vi "Tidy Project.vi"   [LabVIEW 2018]
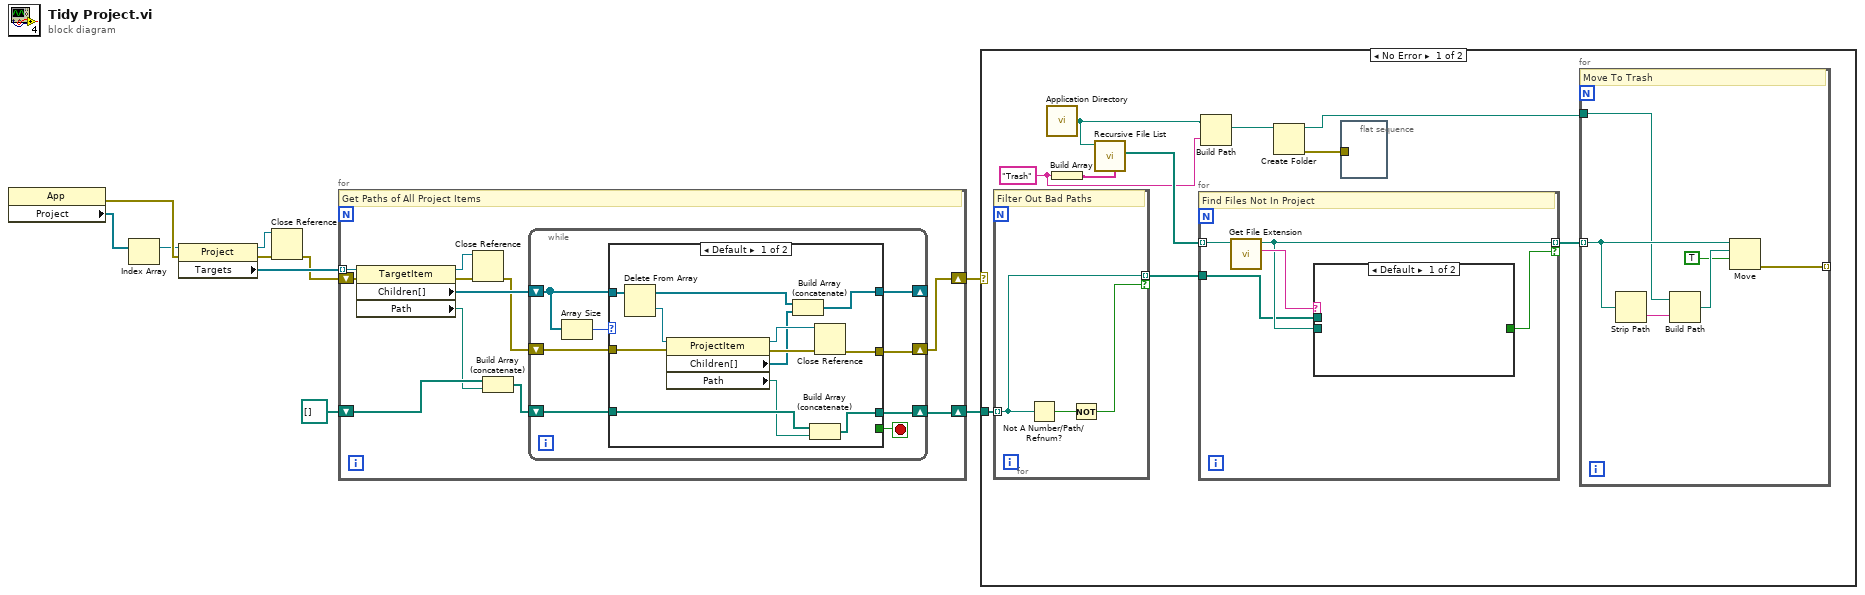
[diagram p0: block diagram]
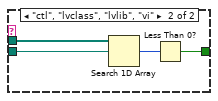
[diagram p2: hidden frame]
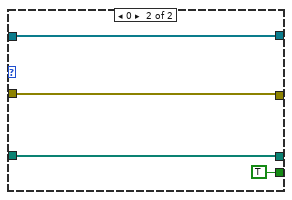
[diagram p4: hidden frame]
diagram:
  n1 = property class="App"() -> (error out=w9:errorcluster, "Project"=w10:refnum<vi>[])  [unwired: 2 in, 1 out]
  n2 = Index Array(array=w10) -> (element=w3:refnum<vi>)  [unwired: 1 in]
  n3 = property class="Project"(reference=w3, error in=w9) -> (reference out=w6:refnum<vi>, error out=w5:errorcluster, "Targets"=w8:refnum<vi>[])
  n4 = Close Reference(reference=w6, error in (no error)=w5) -> (error out=w4:errorcluster)
  n5 = for {
    tunnel: w8 -> [w21] mode=indexing
    shift-right: [w11] -> w2
    shift-left: path[] [] -> [w18]
    shift-right: [w12] -> w1
    shift-left: w4 -> [w19]
    # "Get Paths of All Project Items"
    n6 = property class="TargetItem"(reference=w21, error in=w19) -> (reference out=w16:refnum<vi>, error out=w17:errorcluster, "Children[]"=w20:refnum<vi>[], "Path"=w13:path)
    n7 = Close Reference(reference=w16, error in (no error)=w17) -> (error out=w15:errorcluster)
    n8 = Build Array (concatenate)(w18, w13) -> (w14:path[])
    n9 = while {
      shift-right: [w24] -> w12
      shift-left: w15 -> [w26]
      shift-right: [w22] -> _
      shift-left: w20 -> [w27]
      shift-right: [w23] -> w11
      shift-left: w14 -> [w25]
      stop <- w28 stop-if-true
      n10 = Array Size(array=w27) -> (size(s)=w29:i32)
      n11 = case shown="Default" w29 {
        tunnel: [_ TRUE] -> w28
        tunnel: w27 -> [w41 w42]
        tunnel: w26 -> [w38 w44]
        tunnel: w25 -> [w34 w43]
        tunnel: [w35 w44] -> w24
        tunnel: [w33 w43] -> w23
        tunnel: [w32 w42] -> w22
        frame Default {
          n12 = Delete From Array(array=w41) -> (deleted portion=w40:refnum<vi>, array with subset deleted=w39:refnum<vi>[])  [unwired: 2 in]
          n13 = property class="ProjectItem"(reference=w40, error in=w38) -> (reference out=w36:refnum<vi>, error out=w37:errorcluster, "Children[]"=w30:refnum<vi>[], "Path"=w31:path)
          n14 = Build Array (concatenate)(w39, w30) -> (w32:refnum<vi>[])
          n15 = Build Array (concatenate)(w34, w31) -> (w33:path[])
          n16 = Close Reference(reference=w36, error in (no error)=w37) -> (error out=w35:errorcluster)
        }
        frame 0 {
        }
      }
    }
  }
  n17 = case shown="No Error" w1 {
    tunnel: w2 -> [w55 _]
    frame No Error {
      w50 = "Trash" ("String")
      n18 = for {
        tunnel: w55 -> [w73] mode=indexing
        tunnel: [w73] -> w53 mode=indexing if=w71
        # "Filter Out Bad Paths"
        n19 = Not A Number/Path/Refnum?(number/path/refnum=w73) -> (NaN/Path/Refnum?=w72:bool)
        n20 = Not(x=w72) -> (.not. x?=w71:bool)
      }
      n21 = call <vilib>:"Application Directory.vi"() -> ("Application Directory"=w51:path)
      n22 = Build Array(w50) -> (w52:string[])
      n23 = call <vilib>:"Recursive File List.vi"("Folders to Exclude"=w52, "Folder Path"=w51) -> ("All Files in Dir"=w54:path[])  [unwired: 5 in, 4 out]
      n24 = for {
        tunnel: w54 -> [w66] mode=indexing
        tunnel: [w64] -> w49 mode=indexing if=w62
        tunnel: w53 -> [w63]
        # "Find Files Not In Project"
        n25 = call <vilib>:"Get File Extension.vi"("file"=w66) -> ("lowercase file extension"=w65:string, "dup file"=w64:path)  [unwired: 6 in, 3 out]
        n26 = case shown="Default" w65 {
          tunnel: w64 -> [_ w69]
          tunnel: w63 -> [_ w68]
          tunnel: [_ w67] -> w62
          frame Default {
          }
          frame "ctl", "lvclass", "lvlib", "vi" {
            n27 = Search 1D Array(1D array=w68, element=w69) -> (index of element=w70:i32)  [unwired: 1 in]
            n28 = Less Than 0?(x=w70) -> (x < 0?=w67:bool)
          }
        }
      }
      n29 = Build Path(base path=w51, name or relative path=w50) -> (appended path=w48:path)
      n30 = Create Folder(path (use dialog)=w48) -> (created path=w46:path, error out=w47:errorcluster)  [unwired: 2 in, 1 out]
      n31 = flat-sequence {
        tunnel: w47 -> [_]
        frame #0 {
        }
      }
      n32 = for {
        tunnel: w49 -> [w61] mode=indexing
        tunnel: w46 -> [w60]
        tunnel: [w57] -> _ mode=indexing
        # "Move To Trash"
        n33 = Strip Path(path=w61) -> (name=w59:string)  [unwired: 1 out]
        n34 = Build Path(base path=w60, name or relative path=w59) -> (appended path=w58:path)
        n35 = Move(source path=w61, 9:TRUE ("overwrite (F)"), 10:w58) -> (error out=w57:errorcluster)  [unwired: 2 in, 2 out]
      }
    }
    frame Error {
    }
  }
